vi "VD-getDataSet.vi"(8 "error in (no error)":errorcluster, 11 "VD-LV-LiteVNA in":refnum<class "VD-LV-LiteVNA.lvclass">) -> (0 "error out":errorcluster, 1 "Valid Data?":bool, 2 "VNA data":T1, 3 "VD-LV-LiteVNA out":refnum<class "VD-LV-LiteVNA.lvclass">, 4 "data status":T2)   [LabVIEW 2020, in "VD-LV-LiteVNA.lvclass"]
uses:
  VD-LV-LiteVNA.lvclass
  VD-data_read_status.ctl
  VD-VNA_data.ctl
  VD-LV-LiteVNA.lvclass/VD-LV-LiteVNA.ctl
  VD-data_req.ctl
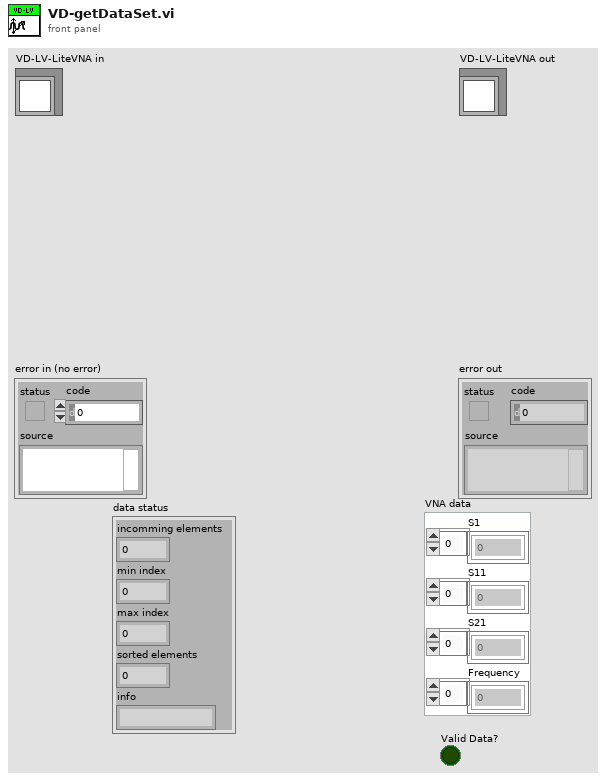
[diagram p1: front panel]
types:
  T1 = typedef "VD-LV-LiteVNA.lvclass/VD-VNA_data.ctl" = cluster{"S1":cdb[], "S11":cdb[], "S21":cdb[], "Frequency":u64[]}
  T2 = typedef "VD-LV-LiteVNA.lvclass/VD-data_read_status.ctl" = cluster{"incomming elements":i32, "min index":u16, "max index":u16, "sorted elements":i32, "info":string}
  T3 = typedef "VD-LV-LiteVNA.lvclass/VD-data_req.ctl" = cluster{"datasize":u8}
  T4 = typedef "HP-S-Serial.lvclass/HP-S-data.ctl" = u8[]
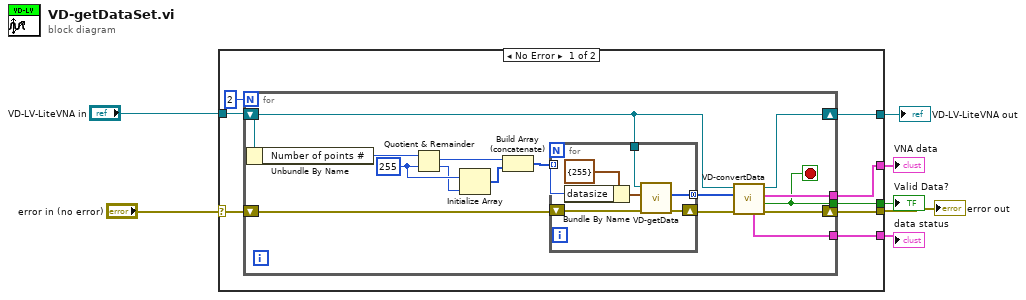
[diagram p0: block diagram]
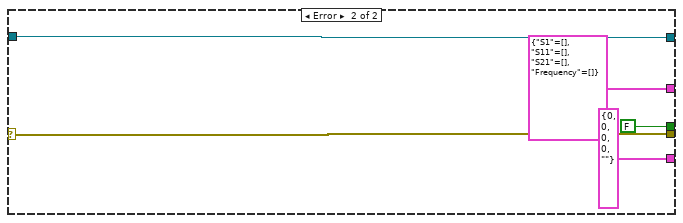
[diagram p2: hidden frame]
diagram:
  n1 = case shown="No Error" "error in (no error)" {
    selector: "error in (no error)" -> [w15 w42]
    tunnel: [w13 w42] -> w6
    tunnel: [w12 w41] -> w4
    tunnel: "VD-LV-LiteVNA in" -> [w14 w41]
    tunnel: [w11 FALSE ("Valid Data?")] -> w3
    tunnel: [w10 T2 {"incomming elements"=0, "min index"=0, "max index"=0, "sorted elements"=0, "info"=""} ("data status")] -> w2
    tunnel: [w9 T1 {"S1"=[], "S11"=[], "S21"=[], "Frequency"=[]} ("VNA data")] -> w1
    frame No Error {
      n2 = for {
        N: 2 -> [_]
        tunnel: [w16] -> w11
        tunnel: [w22] -> w10
        tunnel: [w21] -> w9
        shift-right: [w24] -> w13
        shift-left: w15 -> [w29]
        shift-right: [w23] -> w12
        shift-left: w14 -> [w27]
        stop <- w16 stop-if-true
        w20 = u16 255 ("y")
        n3 = Unbundle By Name(w27) -> ("Number of points #"=w30:u16)
        n4 = Quotient & Remainder(x=w30, y=w20) -> (x-y*floor(x/y)=w17:u16, floor(x/y)=w19:u16)
        n5 = Initialize Array(w20, w19) -> (w18:u16[])
        n6 = Build Array (concatenate)(w17, w18) -> (w28:u16[])
        n7 = for {
          tunnel: w27 -> [w36]
          tunnel: [w35] -> w26 mode=concatenating
          shift-right: [w34] -> w25
          shift-left: w29 -> [w33]
          tunnel: w28 -> [w31] mode=indexing
          n8 = Bundle By Name(cluster=T3 {"datasize"=255} ("data req"), "datasize"=w31) -> (w32:T3)
          n9 = call-dynamic "VD-getData.vi"("error in (no error)"=w33, "data req"=w32, "VD-LV-LiteVNA in"=w36) -> ("error out"=w34:errorcluster, "read buffer"=w35:T4)  [unwired: 6 in, 1 out]
        }
        n10 = call-dynamic "VD-convertData.vi"("error in (no error)"=w25, "read buffer"=w26, "VD-LV-LiteVNA in"=w27) -> ("error out"=w24:errorcluster, "Valid Data?"=w16:bool, "VNA data"=w21:T1, "VD-LV-LiteVNA out"=w23:refnum<class "VD-LV-LiteVNA.lvclass">, "data status"=w22:T2)  [unwired: 4 in]
      }
    }
    frame Error {
    }
  }
  "error out" <- w6
  "VD-LV-LiteVNA out" <- w4
  "Valid Data?" <- w3
  "data status" <- w2
  "VNA data" <- w1
